vi "source Write.vi"(4 "error in (no error)":errorcluster, 5 "Value":T2, 6 "Container State":T5, 7 "Display State In":T3={"SP_Source"={"connect"=FALSE, "SP_Source"=enum."initialize", "SP_Set"=0.0, "SP"=0.0}, "Write"=FALSE, "button state"=enum."init", "reset_timer"=FALSE, "load_timer"=FALSE, "Time"=0, "t ms"=0, "tick"=0, "scale maximum"=100.0}) -> (0 "error out":errorcluster, 3 "Display State Out":T3={"SP_Source"={"connect"=FALSE, "SP_Source"=enum."initialize", "SP_Set"=0.0, "SP"=0.0}, "Write"=FALSE, "button state"=enum."init", "reset_timer"=FALSE, "load_timer"=FALSE, "Time"=0, "t ms"=0, "tick"=0, "scale maximum"=100.0})   [LabVIEW 2019, in "control.lvlib" / "SP_h1.xctl"]
uses:
  SP_h1.xctl
  <vilib>/_xctls/Container State.ctl
  State.ctl
  Heating/ctl/Y_source.ctl
  Y_controlState.ctl
  <vilib>/_xctls/XControlSupport.lvlib
  Heating/Heating.lvlib
panel:
  # "Replace the Value Control below with a Control of desired type.\nDo not remove this Control or the others from the connector pane.\nDo not change the connector pane pattern.\nThe Value control should always be the third terminal from top on the input side in the connector pane."
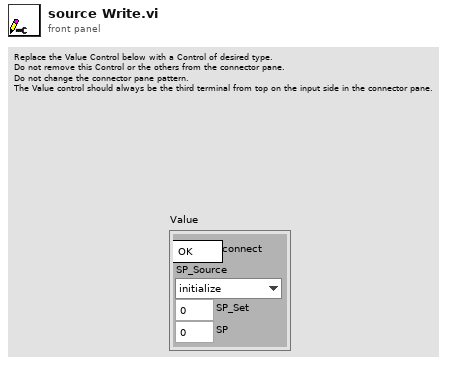
[diagram p1: front panel]
types:
  T1 = typedef "Heating.lvlib/Y_source.ctl" = enum8{"initialize", "local disabled", "local hand", "hand", "auto", "dist"}
  T2 = cluster{"connect":bool, "SP_Source":T1, "SP_Set":dbl, "SP":dbl}
  T3 = typedef "control.lvlib/SP_h1.xctl/State.ctl" = cluster{"SP_Source":cluster{"connect":bool, "SP_Source":T1, "SP_Set":dbl, "SP":dbl}, "Write":bool, "button state":T4, "reset_timer":bool, "load_timer":bool, "Time":u32, "t ms":u32, "tick":u32, "scale maximum":dbl}
  T4 = typedef "control.lvlib/SP_h1.xctl/Y_controlState.ctl" = enum16{"init", "not connect", "local disabled", "local hand", "hand", "value change", "auto", "dist"}
  T5 = typedef "XControlSupport.lvlib/Container State.ctl" = cluster{"Indicator?":bool, "Run Mode?":bool, " Refnum":refnum<vi>}
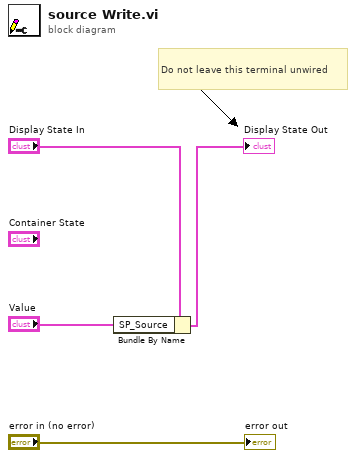
[diagram p0: block diagram]
diagram:
  # "Do not leave this terminal unwired"
  n1 = Bundle By Name(cluster="Display State In", "SP_Source"="Value") -> (→"Display State Out":T3)
  "error out" <- "error in (no error)"
